vi "Transition Measurements (obs).vi"   [LabVIEW 2020, in "NI_MAPro.lvlib"]
uses:
  NI_MAPro.lvlib
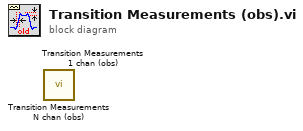
[diagram p0: block diagram]
diagram:
  n1 = call "Transition Measurements N chan (obs).vi"() -> ()  [unwired: 6 in, 6 out]
  n2 = call "Transition Measurements 1 chan (obs).vi"() -> ()  [unwired: 6 in, 6 out]
